vi "Drive_Globals.vi"() -> ()   [LabVIEW 2018]
uses:
  Subsytems/Drive/Drive_Notifier.ctl
  Subsytems/Drive/Drive_Control_Type.ctl
panel:
  out "Algorithm_Enable":bool
  out "Zero_Front_Right":bool
  out "Zero_Back_Right":bool
  out "Zero_Back_Left":bool
  out "Zero_Wheels_Btn_Pressed":bool
  in  "Pigeon_IMU_2":string="Pigeon_IMU_2"
  in  "Pigeon_IMU_1":string="Pigeon_IMU_1"
  out "Zero_Front_Left":bool
  in  "Drive_Execute_Notifier":string="Drive_Execute_Notifier"
  in  "Drive_Set_Notifier":string="Drive_Set_Notifier"
  in  "BR_Limit":string="Back Right Limit"
  in  "BL_Limit":string="Back Left Limit"
  in  "FR_Limit":string="Front Right Limit"
  in  "FL_Limit":string="Front Left Limit"
  in  "BR_Zero":dbl=2211.0
  in  "BL_Zero":dbl=2256.0
  in  "FR_Zero":dbl=3740.0
  in  "FL_Zero":dbl
  in  "BR_Init":dbl=-1095.0
  in  "BL_Init":dbl=-818.0
  in  "FR_Init":dbl=-924.0
  in  "FL_Init":dbl=-1370.0
  in  "Drive_Execute_Ref":refnum<notifier>
  in  "Back_Right_Steer":string="Right Back Wheel Spin"
  in  "Front_Right_Steer":string="Right Front Wheel Spin"
  in  "Front_Left_Steer":string="Left Front Wheel Spin"
  in  "Back_Left_Steer":string="Left Back Wheel Spin"
  in  "Back_Right_Drive":string="Right Back Wheel Drive"
  in  "Front_Right_Drive":string="Right Front Wheel Drive"
  in  "Front_Left_Drive":string="Left Front Wheel Drive"
  in  "Back_Left_Drive":string="Left Back Wheel Drive"
  in  "Drive_Set_Ref":refnum<notifier>
  # "s"
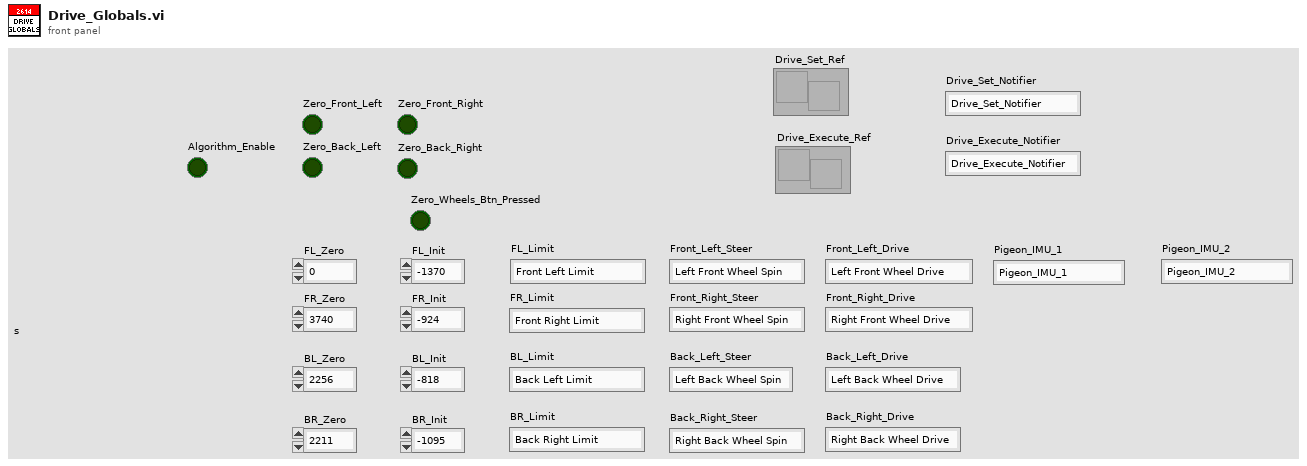
[diagram p1: front panel]
diagram:
